vi "Eagle_FPGA Ranging Beams Intensity.vi"() -> ()   [LabVIEW 2015]
uses:
  <vilib>/rvi/Emulation/niFpgaGetClockAttributes.vi
  <vilib>/rvi/Emulation/niFpgaSctlEmulationGetInTimedLoop.vi
  <vilib>/rvi/Emulation/niFpgaEmulationReportErrorSimple.vi
  <vilib>/rvi/eio/common/nirviEmuTemplateMethod_errors.vi
  <vilib>/rvi/Emulation/niFpgaCriticalErrorInLSC.vi
  <vilib>/eio/EIONode/EIONode.xnode
panel:
  in  "RB Intensity":fxp<+,16,3>
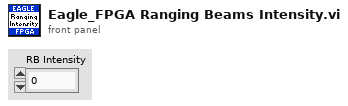
[diagram p1: front panel]
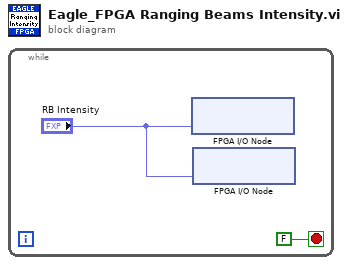
[diagram p0: block diagram]
diagram:
  n1 = while {
    stop <- FALSE stop-if-true
    n2 = xnode "FPGA I/O Node"("Mod3/AO4"="RB Intensity") -> ()  [unwired: 1 in, 1 out]
    n3 = xnode "FPGA I/O Node"("Mod3/AO5"="RB Intensity") -> ()  [unwired: 1 in, 1 out]
  }
